vi "Helper Loop Create.vi"(10 "Helper Loop":refnum<class "Helper Loop.lvclass">, 11 "Panel Create in":refnum<class "Helper Loop Create.lvclass">) -> (3 "Panel Create out":refnum<class "Helper Loop Create.lvclass">)   [LabVIEW 2021, in "Helper Loop Create.lvlib" / "Helper Loop Create.lvclass"]
uses:
  Helper Loop Create.lvclass
  Helper Loop/Helper Loop.lvclass
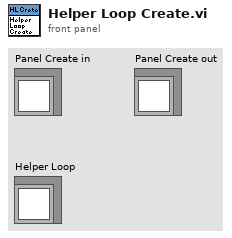
[diagram p1: front panel]
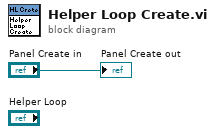
[diagram p0: block diagram]
diagram:
  "Panel Create out" <- "Panel Create in"
